vi "Write refs_controls_V0_VD2.vi"(8 "error in (no error)":errorcluster, 9 "EXP":bool=TRUE caption="EXP V0/VD2", 10 "refs_controls_V0":refnum<vi>[](array[refnum]), 11 "Control-Client in":refnum<class "Control-Client.lvclass">) -> (0 "error out":errorcluster, 3 "Control-Client out":refnum<class "Control-Client.lvclass">)   [LabVIEW 2019, in "Control-Client.lvclass"]
uses:
  Control-Client.lvclass
  Control-Client.lvclass/Control-Client.ctl
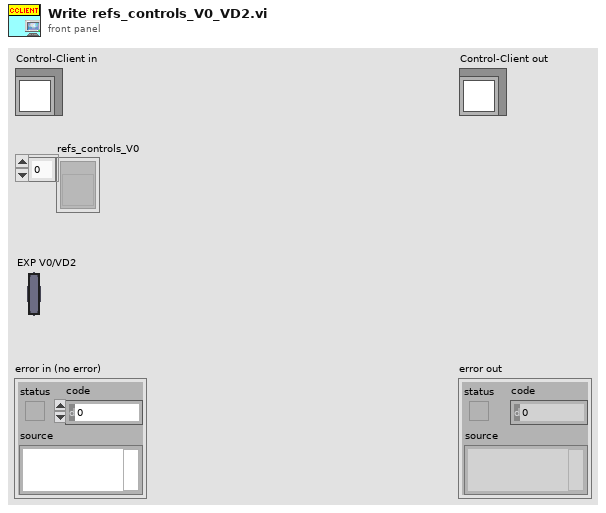
[diagram p1: front panel]
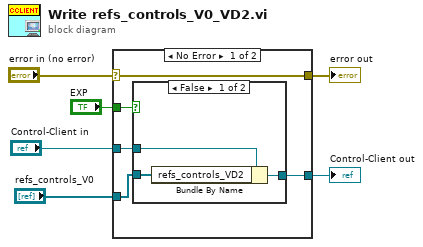
[diagram p0: block diagram]
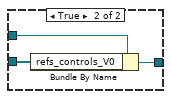
[diagram p2: hidden frame]
diagram:
  n1 = case shown="No Error" "error in (no error)" {
    selector: "error in (no error)" -> [w11 w18]
    tunnel: [w11 w18] -> w5
    tunnel: [w9 w19] -> w3
    tunnel: "Control-Client in" -> [w10 w19]
    tunnel: "refs_controls_V0" -> [w8 _]
    tunnel: "EXP" -> [w7 _]
    frame No Error {
      n2 = case shown="False" w7 {
        tunnel: w10 -> [w13 w17]
        tunnel: [w14 w16] -> w9
        tunnel: w8 -> [w12 w15]
        frame False {
          n3 = Bundle By Name(cluster=w13, "refs_controls_VD2"=w12) -> (w14:refnum<class "Control-Client.lvclass">)
        }
        frame True {
          n4 = Bundle By Name(cluster=w17, "refs_controls_V0"=w15) -> (w16:refnum<class "Control-Client.lvclass">)
        }
      }
    }
    frame Error {
    }
  }
  "error out" <- w5
  "Control-Client out" <- w3
